vi "Read Default Rectangle Cluster.vi"(8 "error in (no error)":errorcluster, 11 "Rectangle Settings in":refnum<class "Rectangle Settings.lvclass">) -> (0 "error out":errorcluster, 2 "Default Rectangle Cluster":T1, 3 "Rectangle Settings out":refnum<class "Rectangle Settings.lvclass">)   [LabVIEW 2019, in "Rectangle Settings.lvclass"]
uses:
  Rectangle Settings.lvclass
  Typedefs/Default Rectangle Cluster.ctl
  Rectangle Settings.lvclass/Rectangle Settings.ctl
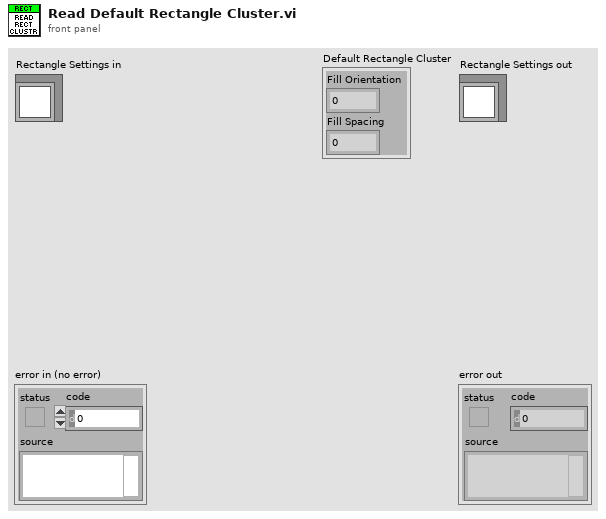
[diagram p1: front panel]
types:
  T1 = typedef "Rectangle Settings.lvclass/Default Rectangle Cluster.ctl" = cluster{"Fill Orientation":u16, "Fill Spacing":dbl}
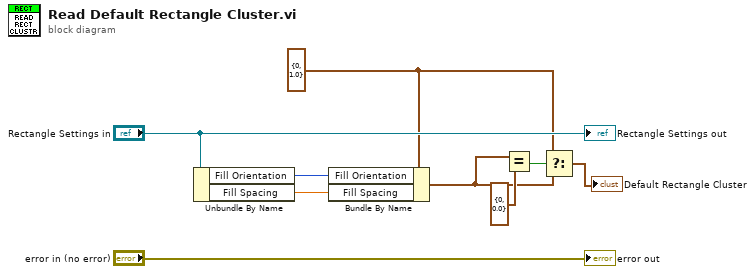
[diagram p0: block diagram]
diagram:
  w4 = T1 {"Fill Orientation"=0, "Fill Spacing"=1.0} ("cluster")
  n1 = Unbundle By Name("Rectangle Settings in") -> ("Fill Orientation"=w7:u16, "Fill Spacing"=w6:dbl)
  n2 = Bundle By Name(cluster=w4, "Fill Orientation"=w7, "Fill Spacing"=w6) -> (w2:T1)
  n3 = Equal?(x=w2, y=T1 {"Fill Orientation"=0, "Fill Spacing"=0.0} ("output cluster")) -> (x = y?=w3:bool)
  n4 = Select(t=w4, s=w3, f=w2) -> (s? t:f=→"Default Rectangle Cluster":T1)
  "error out" <- "error in (no error)"
  "Rectangle Settings out" <- "Rectangle Settings in"
